vi "NI VeriStand - Enable System Explorer Update Buffer.vi"(8 "error in (no error)":errorcluster) -> (0 "error out":errorcluster)   [LabVIEW 2020, in "Custom Device API.lvlib"]
doc: "Enables the buffer for updates to the <B>System Explorer</B> window. Using this VI together with the Commit System Explorer Update Buffer VI can speed up item creation if you are creating or updating multiple custom device items at one time."
uses:
  <vilib>/NI VeriStand/Custom Device API/Custom Device API.lvlib
  a86f2752-8446-4cd1-a573-1c8610072916.vi
  <vilib>/NI VeriStand/Custom Device API/Custom Device Offline Path.vi
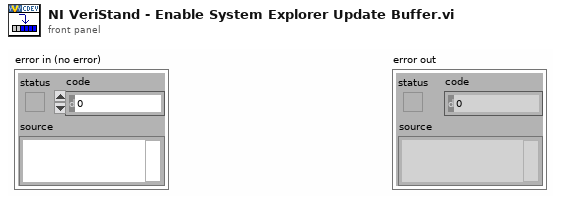
[diagram p1: front panel]
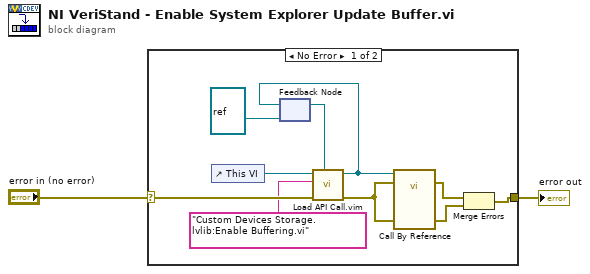
[diagram p0: block diagram]
diagram:
  n1 = case shown="No Error" "error in (no error)" {
    selector: "error in (no error)" -> [w8 w13]
    tunnel: [w11 w13] -> w2
    frame No Error {
      n2 = control-ref of="This VI"() -> (w9:refnum<vi>)
      n3 = feedback #1(refnum<vi> refnum ("type specifier VI Refnum (for type only)")) -> (w10:refnum<vi>)
      n4 = call "Load API Call.vim"("VI reference in"=w10, "error in (no error)"=w8, "VI qualified name"="Custom Devices Storage.lvlib:Enable Buffering.vi", "Caller VI ref"=w9) -> ("error out"=w7:errorcluster, "VI reference"=w6:refnum<vi>)  [unwired: 6 in]
      n5 = feedback-in #1(w6) -> ()
      n6 = call-by-ref "?"(reference=w6, error in=w7, 8:"error in (no error)"=w7) -> (error out=w3:errorcluster, 0:"error out"=w12:errorcluster)  [unwired: 10 in, 1 out]
      n7 = Merge Errors(w3, w12) -> (w11:errorcluster)
    }
    frame Error {
    }
  }
  "error out" <- w2
